vi "SV Converter.vi"(4 "SV":refnum<k21>) -> (1 "AEgIS Shared Variables out":refnum<class "Circus Shared Variables.lvclass">)   [LabVIEW 2026, in "TALOS.lvlib" / "Classes.lvlib" / "Circus Shared Variables.lvclass"]
doc: "Use this VI to convert a Shared Variable to an AEgIS Shared Variable. For legacy support."
uses:
  Circus Shared Variables.lvclass
  Circus Shared Variables.lvclass/Circus Shared Variables.ctl
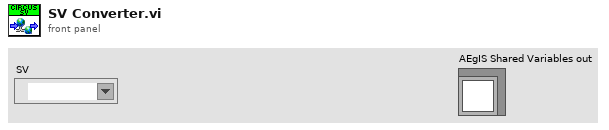
[diagram p1: front panel]
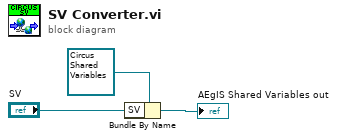
[diagram p0: block diagram]
diagram:
  n1 = Bundle By Name(cluster=refnum<class "Circus Shared Variables.lvclass"> refnum ("AEgIS Shared Variables out"), "SV"="SV") -> (→"AEgIS Shared Variables out":refnum<class "Circus Shared Variables.lvclass">)
